vi "calcolo_coefficienti.vi"(0 "Reali":cluster{"Re1":dbl, "Re2":dbl}, 1 "Coefficienti":cluster{"A":i16, "B":i16, "C":i16}) -> ()   [LabVIEW 2022 SP3]
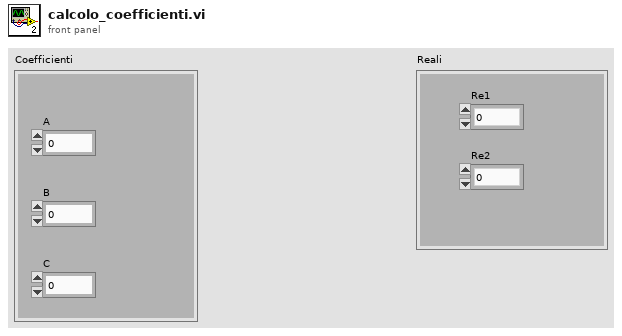
[diagram p1: front panel]
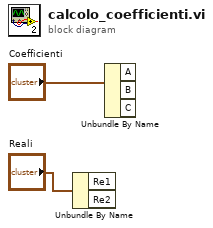
[diagram p0: block diagram]
diagram:
  n1 = Unbundle By Name("Reali") -> ()  [unwired: 2 out]
  n2 = Unbundle By Name("Coefficienti") -> ()  [unwired: 3 out]
